vi "Measure (Hardcoded Dependency).vi"(10 "t":dbl, 11 "Sine in":refnum<class "Sine.lvclass">) -> (2 "y":dbl)   [LabVIEW 2024]
uses:
  Classes/Sine/Sine.lvclass
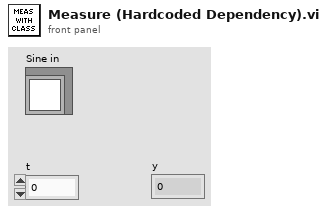
[diagram p1: front panel]
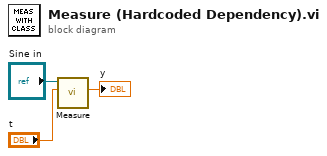
[diagram p0: block diagram]
diagram:
  n1 = call-dynamic "Measure.vi"("t (seconds)"="t", "Sine in"="Sine in") -> ("y"=→"y":dbl)  [unwired: 8 in, 1 out]
